vi "New.vi"(10 "DMM.lvclass":refnum<class "DMM.lvclass">, 11 "Keysight.lvclass":refnum<class "Keysight.lvclass">) -> (3 "output cluster":refnum<class "DMMArray.lvclass">)   [LabVIEW 2020, in "DMMArray.lvclass"]
uses:
  DMMArray.lvclass
  Keysight/Keysight.lvclass
  C:/Repo/LabVIEW-SOLID-Examples/SOLID-Dataflow-Template/IReference/IDMM.lvclass
  DMM/DMM.lvclass
  DMMArray.lvclass/DMMArray.ctl
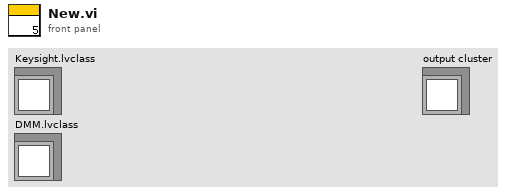
[diagram p1: front panel]
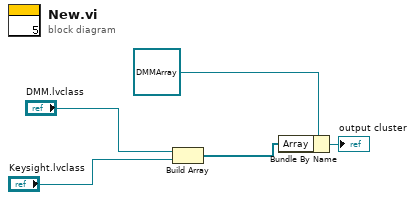
[diagram p0: block diagram]
diagram:
  n1 = Build Array("DMM.lvclass", "Keysight.lvclass") -> (w2:refnum<class "IDMM.lvclass">[])
  n2 = Bundle By Name(cluster=refnum<class "DMMArray.lvclass"> refnum ("DMMArray.lvclass"), "Array"=w2) -> (→"output cluster":refnum<class "DMMArray.lvclass">)
